vi "Define Master Slave Relationship.vi"(4 "error in (no error)":errorcluster, 5 "Master Axis":i32=1 min=1 max=3, 6 "Slave Axis":i32=1 min=1 max=3, 7 "VISA resource name":refnum<visa-resource-name>) -> (0 "error out":errorcluster, 3 "VISA resource name out":refnum<visa-resource-name>)   [LabVIEW 2018, in "Newport ESP301.lvlib"]
doc: "This command defines master-slave relationship between any two axes. A few rules are in place for ease of use.\n1) The trajectory mode for slave has to be appropriately defined before that axis follows master in a desired fashion.\n2) An axis cannot be assigned as its own slave if it is already in a trajectory mode that is specific to master-slaving.\n3) A slave axis cannot be moved individually using PA or PR commands if its trajectory mode is specific to master-slaving.\nThis command gets executed immediately, and can also be called from within a program."
uses:
  Newport ESP301.lvlib
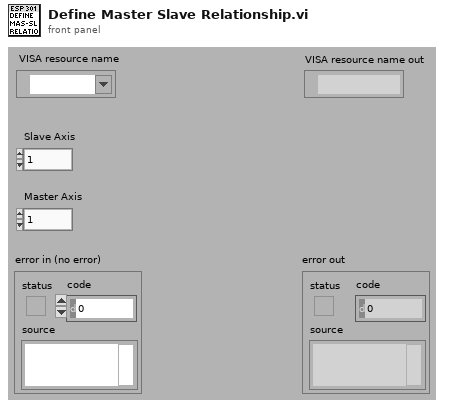
[diagram p1: front panel]
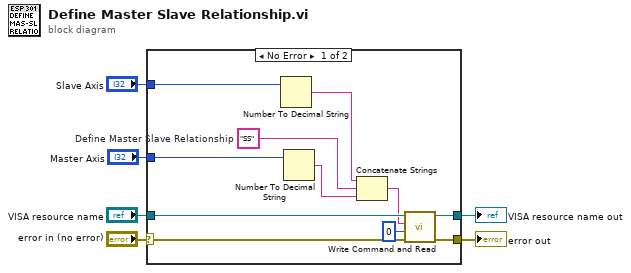
[diagram p0: block diagram]
diagram:
  n1 = case shown="No Error" "error in (no error)" {
    selector: "error in (no error)" -> [w16 w19]
    tunnel: [w15 w19] -> w6
    tunnel: "VISA resource name" -> [w17 w18]
    tunnel: [w14 w18] -> w5
    tunnel: "Slave Axis" -> [w11 _]
    tunnel: "Master Axis" -> [w8 _]
    frame No Error {
      w12 = "SS"  # Define Master Slave Relationship
      n2 = Number To Decimal String(number=w11) -> (decimal integer string=w13:string)  [unwired: 1 out]
      n3 = Number To Decimal String(number=w8) -> (decimal integer string=w7:string)  [unwired: 1 out]
      n4 = Concatenate Strings(w13, w12, w7) -> (w10:string)
      n5 = call "Write Command and Read.vi"("error in (no error)"=w16, "Bytes to read (100)"=u32 0, "Command"=w10, "VISA resource name"=w17) -> ("error out"=w15:errorcluster, "VISA resource name out"=w14:refnum<visa-resource-name>)  [unwired: 1 in, 3 out]
    }
    frame Error {
    }
  }
  "error out" <- w6
  "VISA resource name out" <- w5
